vi "bandpass_kHz.vi"(8 "Highpass cut (kHz)":dbl, 9 "Lowpass cut (kHz)":dbl, 10 "dt":dbl, 11 "Signal in":dbl[](array[numeric])) -> (1 "Peak2peak(mV)":dbl, 3 "Signal out":dbl[](array[numeric]))   [LabVIEW 2016]
uses:
  <vilib>/Analysis/3filter.llb/Filter Passband Type.ctl
  <vilib>/Analysis/3filter.llb/Butterworth Filter (DBL).vi
  <vilib>/Analysis/NI_AALBase.lvlib
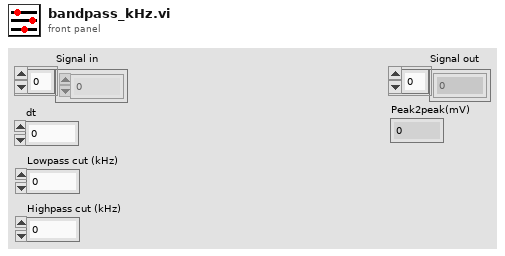
[diagram p1: front panel]
types:
  T1 = typedef "NI_AALBase.lvlib/Filter Passband Type.ctl" = enum32{"Lowpass", "Highpass", "Bandpass", "Bandstop"}
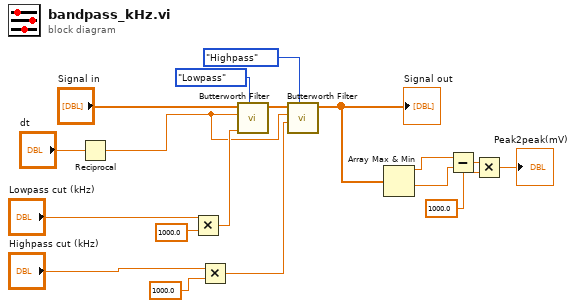
[diagram p0: block diagram]
diagram:
  n1 = Reciprocal(x="dt") -> (1/x=w10:dbl)
  n2 = Multiply(x="Lowpass cut (kHz)", y=1000.0 ("low cutoff freq: fl")) -> (x*y=w16:dbl)
  n3 = Multiply(x="Highpass cut (kHz)", y=1000.0 ("low cutoff freq: fl")) -> (x*y=w8:dbl)
  n4 = call-poly <vilib>:"Butterworth Filter.vi"("filter type"=Filter_Passband_Type."Lowpass", "low cutoff freq: fl"=w16, "sampling freq: fs"=w10, "X"="Signal in") -> ("Filtered X"=w15:dbl[])  [unwired: 4 in, 1 out]
  n5 = call-poly <vilib>:"Butterworth Filter.vi"("filter type"=Filter_Passband_Type."Highpass", "high cutoff freq: fh"=w8, "sampling freq: fs"=w10, "X"=w15) -> ("Filtered X"=w2:dbl[])  [unwired: 4 in, 1 out]
  "Signal out" <- w2
  n6 = Array Max & Min(array=w2) -> (max value=w6:dbl, min value=w5:dbl)  [unwired: 2 out]
  n7 = Subtract(x=w6, y=w5) -> (x-y=w3:dbl)
  n8 = Multiply(x=w3, y=1000.0) -> (x*y=→"Peak2peak(mV)":dbl)
